vi "Get Parameters Indexes.vi"(8 "error in":errorcluster, 11 "data dictionary in":refnum<class "data dictionary.lvclass">) -> (0 "error out":errorcluster, 2 "Parameter Indexes":T1)   [LabVIEW 2015, in "Sequencer Module tests.lvlib"]
uses:
  Sequencer Module tests.lvlib
  <vilib>/NI/Tag Bus/dictionary/data dictionary.lvclass
  Parameters Indexes.ctl
  <vilib>/NI/Tag Bus/dictionary/data dictionary.lvclass/data dictionary.ctl
  <vilib>/NI/Tag Bus/dictionary/lookup polymorphs/locate Boolean.vi
  <vilib>/NI/Tag Bus/dictionary/lookup polymorphs/locate String.vi
  <vilib>/NI/Tag Bus/dictionary/search/find data index.vi
  <vilib>/NI/Tag Bus/dictionary/search/search string list.vi
  <vilib>/NI/Tag Bus/dictionary/tag not found.vi
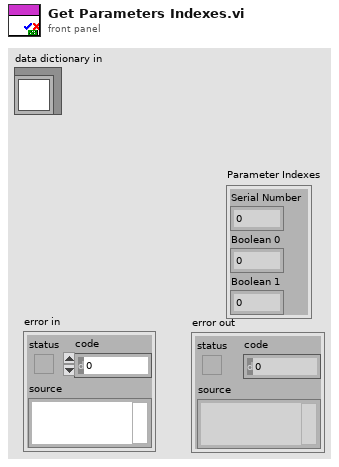
[diagram p1: front panel]
types:
  T1 = typedef "Parameters Indexes.ctl" = cluster{"Serial Number":i32, "Boolean 0":i32, "Boolean 1":i32}
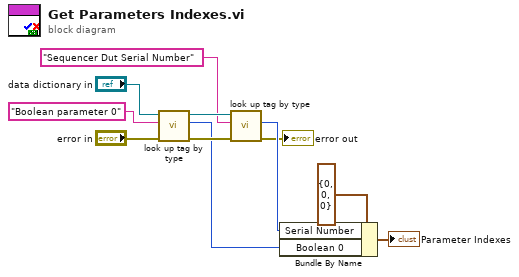
[diagram p0: block diagram]
diagram:
  n1 = call-poly <vilib>:"look up tag by type.vi"("error in"="error in", "name"="Boolean parameter 0", "data dictionary in"="data dictionary in") -> ("error out"=w11:errorcluster, "index"=w3:i32, "data dictionary out"=w10:refnum<class "data dictionary.lvclass">)  [unwired: 6 in]
  n2 = call-poly <vilib>:"look up tag by type.vi"("error in"=w11, "name"="Sequencer Dut Serial Number", "data dictionary in"=w10) -> ("error out"=→"error out":errorcluster, "index"=w5:i32)  [unwired: 6 in, 1 out]
  n3 = Bundle By Name(cluster=T1 {"Serial Number"=0, "Boolean 0"=0, "Boolean 1"=0} ("Parameter Indexes"), "Serial Number"=w5, "Boolean 0"=w3) -> (→"Parameter Indexes":T1)
